vi "Cholesky Factorization Rank-1 Update_Givens Rotation (DBL).vi"(10 "b":dbl, 11 "a":dbl) -> (1 "v":dbl, 2 "s":dbl, 3 "c":dbl)   [LabVIEW 2020, in "NI_AAL_LinAlg.lvlib"]
uses:
  <vilib>/Analysis/NI_AAL_LinAlg.lvlib
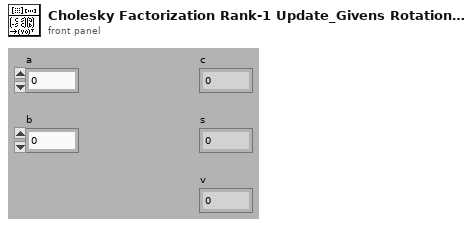
[diagram p1: front panel]
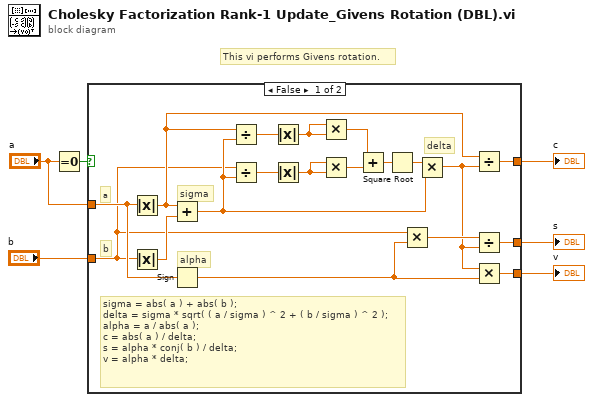
[diagram p0: block diagram]
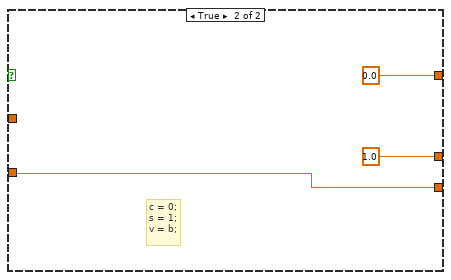
[diagram p2: hidden frame]
diagram:
  # "This vi performs Givens rotation."
  n1 = Equal To 0?(x="a") -> (x = 0?=w6:bool)
  n2 = case shown="False" w6 {
    tunnel: "b" -> [w7 w27]
    tunnel: "a" -> [w8 _]
    tunnel: [w19 0.0] -> w3
    tunnel: [w17 1.0] -> w2
    tunnel: [w16 w27] -> w1
    frame False {
      # "alpha"
      # "b"
      # "a"
      # "delta"
      # "sigma"
      # "sigma = abs( a ) + abs( b );\ndelta = sigma * sqrt( ( a / sigma ) ^ 2 + ( b / sigma ) ^ 2 );\nalpha = a / abs( a );\nc = abs( a ) / delta;\ns = alpha * conj( b ) / delta;\nv = alpha * delta;"
      n3 = Absolute Value(x=w8) -> (abs(x)=w10:dbl)
      n4 = Absolute Value(x=w7) -> (abs(x)=w25:dbl)
      n5 = Add(x=w10, y=w25) -> (x+y=w20:dbl)
      n6 = Sign(1:w8) -> (0:w9:dbl)
      n7 = Divide(x=w10, y=w20) -> (x/y=w14:dbl)
      n8 = Divide(x=w7, y=w20) -> (x/y=w12:dbl)
      n9 = Absolute Value(x=w14) -> (abs(x)=w13:dbl)
      n10 = Absolute Value(x=w12) -> (abs(x)=w11:dbl)
      n11 = Multiply(x=w13, y=w13) -> (x*y=w23:dbl)
      n12 = Multiply(x=w11, y=w11) -> (x*y=w24:dbl)
      n13 = Add(x=w23, y=w24) -> (x+y=w22:dbl)
      n14 = Square Root(x=w22) -> (sqrt(x)=w21:dbl)
      n15 = Multiply(x=w7, y=w9) -> (x*y=w18:dbl)
      n16 = Multiply(x=w21, y=w20) -> (x*y=w15:dbl)
      n17 = Divide(x=w10, y=w15) -> (x/y=w19:dbl)
      n18 = Divide(x=w18, y=w15) -> (x/y=w17:dbl)
      n19 = Multiply(x=w15, y=w9) -> (x*y=w16:dbl)
    }
    frame True {
      # "c = 0;\ns = 1;\nv = b;"
    }
  }
  "c" <- w3
  "s" <- w2
  "v" <- w1
